vi "Valve_open.vi"(8 "data":bool[](array[boolean]), 11 "lines":tag) -> (3 "task out":refnum<k21>)   [LabVIEW 2016]
uses:
  <vilib>/DAQmx/write.llb/DAQmx Write (Digital 1D Bool NChan 1Samp 1Line).vi
  <vilib>/DAQmx/create/channels.llb/DAQmx Create Channel (DO-Digital Output).vi
  <vilib>/DAQmx/miscellaneous.llb/DAQmx Fill In Error Info.vi
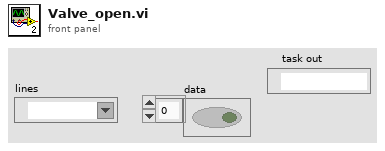
[diagram p1: front panel]
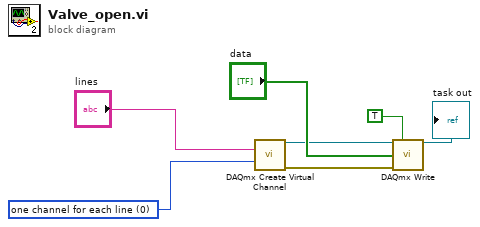
[diagram p0: block diagram]
diagram:
  w3 = 0 items=["one channel for each line", "one channel for all lines"] ("line grouping")
  n1 = call-poly <vilib>:"DAQmx Create Virtual Channel.vi"("lines"="lines", "line grouping"=w3) -> ("task out"=w4:refnum<k21>, "error out"=w5:errorcluster)  [unwired: 12 in]
  n2 = call-poly <vilib>:"DAQmx Write.vi"("task/channels in"=w4, "auto start"=TRUE, "data"="data", "error in"=w5) -> ("task out"=→"task out":refnum<k21>)  [unwired: 9 in, 2 out]
